vi "baogao3.vi"() -> ()   [LabVIEW 2017]
panel:
  out "k":i32
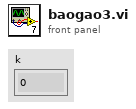
[diagram p1: front panel]
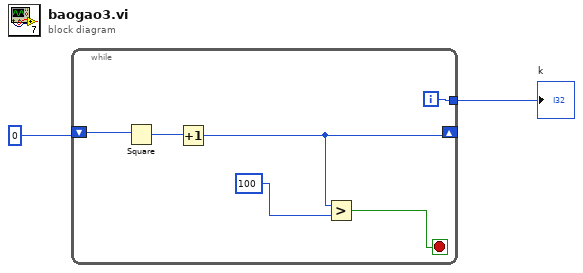
[diagram p0: block diagram]
diagram:
  n1 = while {
    tunnel: [w8] -> w2
    shift-right: [w3] -> _
    shift-left: 0 -> [w7]
    i -> [w8]
    stop <- w4 stop-if-true
    n2 = Square(x=w7) -> (x^2=w6:i32)
    n3 = Increment(x=w6) -> (x+1=w3:i32)
    n4 = Greater?(x=w3, y=100) -> (0:w4:bool)
  }
  "k" <- w2
